vi "main.vi"() -> ()   [LabVIEW 2013]
uses:
  TestMathLib/TestMathLib.lvlib
panel:
  out "Result":dbl(slide) scale=0.0..10.0
  in  "Second Number":dbl(slide) scale=0.0..10.0
  in  "First Number":dbl(slide) scale=0.0..10.0
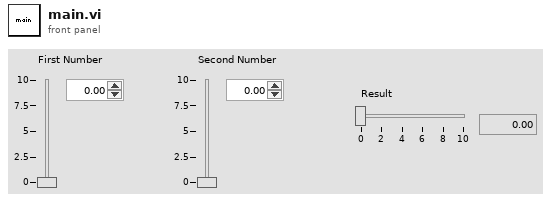
[diagram p1: front panel]
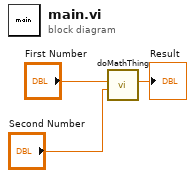
[diagram p0: block diagram]
diagram:
  n1 = call "doMathThing.vi"("Second number"="Second Number", "First number"="First Number") -> ("Result"=→"Result":dbl)  [unwired: 9 in]
